vi "Construct Compound Filter.vi"(8 "error in (no error)":errorcluster, 10 "AND Filters? (Default T, F OR)":bool=TRUE, 11 "Filters":refnum<class "ILogFilter.lvclass">[](array[class])) -> (0 "error out":errorcluster, 3 "Compound Filter out":refnum<class "Compound Filter.lvclass">)   [LabVIEW 2017, in "Compound Filter.lvclass"]
doc: "Construct a compound log filter - inject nested filters to use multiple log filters. Boolean AND Filters input dedicates whether filters will be ANDed or ORed to determine log status."
uses:
  Compound Filter.lvclass
  Composed Log/ILogFilter/ILogFilter.lvclass
  Compound Filter.lvclass/Compound Filter.ctl
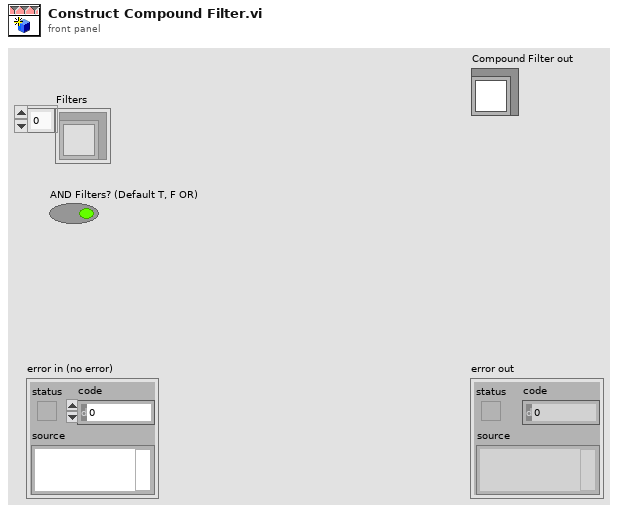
[diagram p1: front panel]
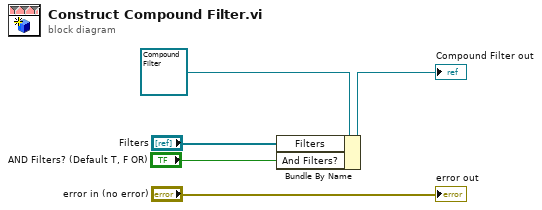
[diagram p0: block diagram]
diagram:
  n1 = Bundle By Name(cluster=refnum<class "Compound Filter.lvclass"> refnum ("Compound Filter in"), "Filters"="Filters", "And Filters?"="AND Filters? (Default T, F OR)") -> (→"Compound Filter out":refnum<class "Compound Filter.lvclass">)
  "error out" <- "error in (no error)"
